vi "Read MERCANCIA.vi"(8 "error in (no error)":errorcluster, 11 "UI_PAPAS_MEX_ESP in":refnum<class "UI_PAPAS_MEX_ESP.lvclass">) -> (0 "error out":errorcluster, 2 "MERCANCIA":refnum<vi>, 3 "UI_PAPAS_MEX_ESP out":refnum<class "UI_PAPAS_MEX_ESP.lvclass">)   [LabVIEW 2019, in "UI_PAPAS_MEX_ESP.lvlib" / "UI_PAPAS_MEX_ESP.lvclass"]
uses:
  UI_PAPAS_MEX_ESP.lvclass
  UI_PAPAS_MEX_ESP.lvclass/UI_PAPAS_MEX_ESP.ctl
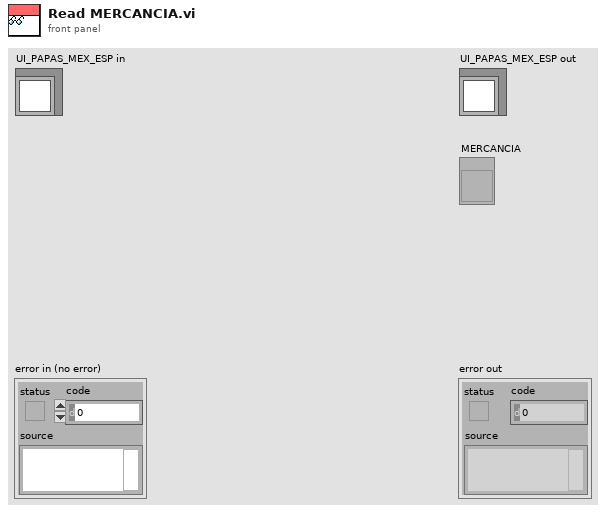
[diagram p1: front panel]
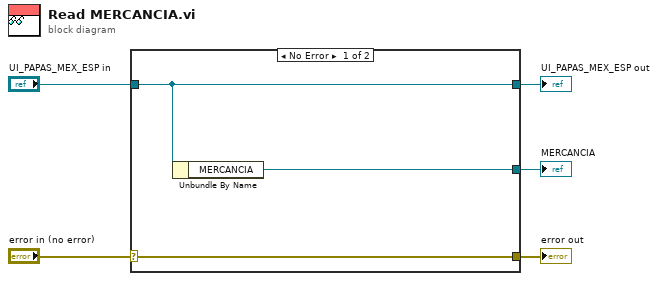
[diagram p0: block diagram]
diagram:
  n1 = case shown="No Error" "error in (no error)" {
    selector: "error in (no error)" -> [w8 w9]
    tunnel: [w8 w9] -> w4
    tunnel: [w7 w10] -> w2
    tunnel: "UI_PAPAS_MEX_ESP in" -> [w7 w10]
    tunnel: [w6 _] -> w1
    frame No Error {
      n2 = Unbundle By Name(w7) -> ("MERCANCIA"=w6:refnum<vi>)
    }
    frame Error {
    }
  }
  "error out" <- w4
  "UI_PAPAS_MEX_ESP out" <- w2
  "MERCANCIA" <- w1
